vi "ArgoBot_Write.vi"(4 "GPIO 3 Write":dbl, 6 "GPIO 2 Write":dbl, 7 "Right Motor":dbl, 8 "Read_Cluster":T8, 9 "GPIO 1 Write":dbl, 10 "LED Write":bool, 11 "Left Motor":dbl) -> (3 "Write Cluster":T7)   [LabVIEW 2016, in "ArgoBotLib.lvlib"]
uses:
  ArgoBotLib.lvlib
  <vilib>/MakerHub/LINX/Private/Type Defs/LINX Ref.ctl
  <vilib>/MakerHub/LINX/Private/Type Defs/Platform.ctl
  <vilib>/MakerHub/LINX/Private/Type Defs/Interface.ctl
  <vilib>/MakerHub/LINX/Private/Device/Type Defs/LINX Device Config.ctl
  <vilib>/MakerHub/LINX/Private/Device/Type Defs/TCP Config.ctl
  <vilib>/MakerHub/LINX/Private/Device/Type Defs/Channels.ctl
  <vilib>/MakerHub/LINX/LMH-LINX.lvlib
  <vilib>/MakerHub/LINX/Private/Device/Device.lvlib
panel:
  # "ArgoBot  Write"
  # "This vi writes the GPIO channels"
  # "Inputs"
  # "Outputs"
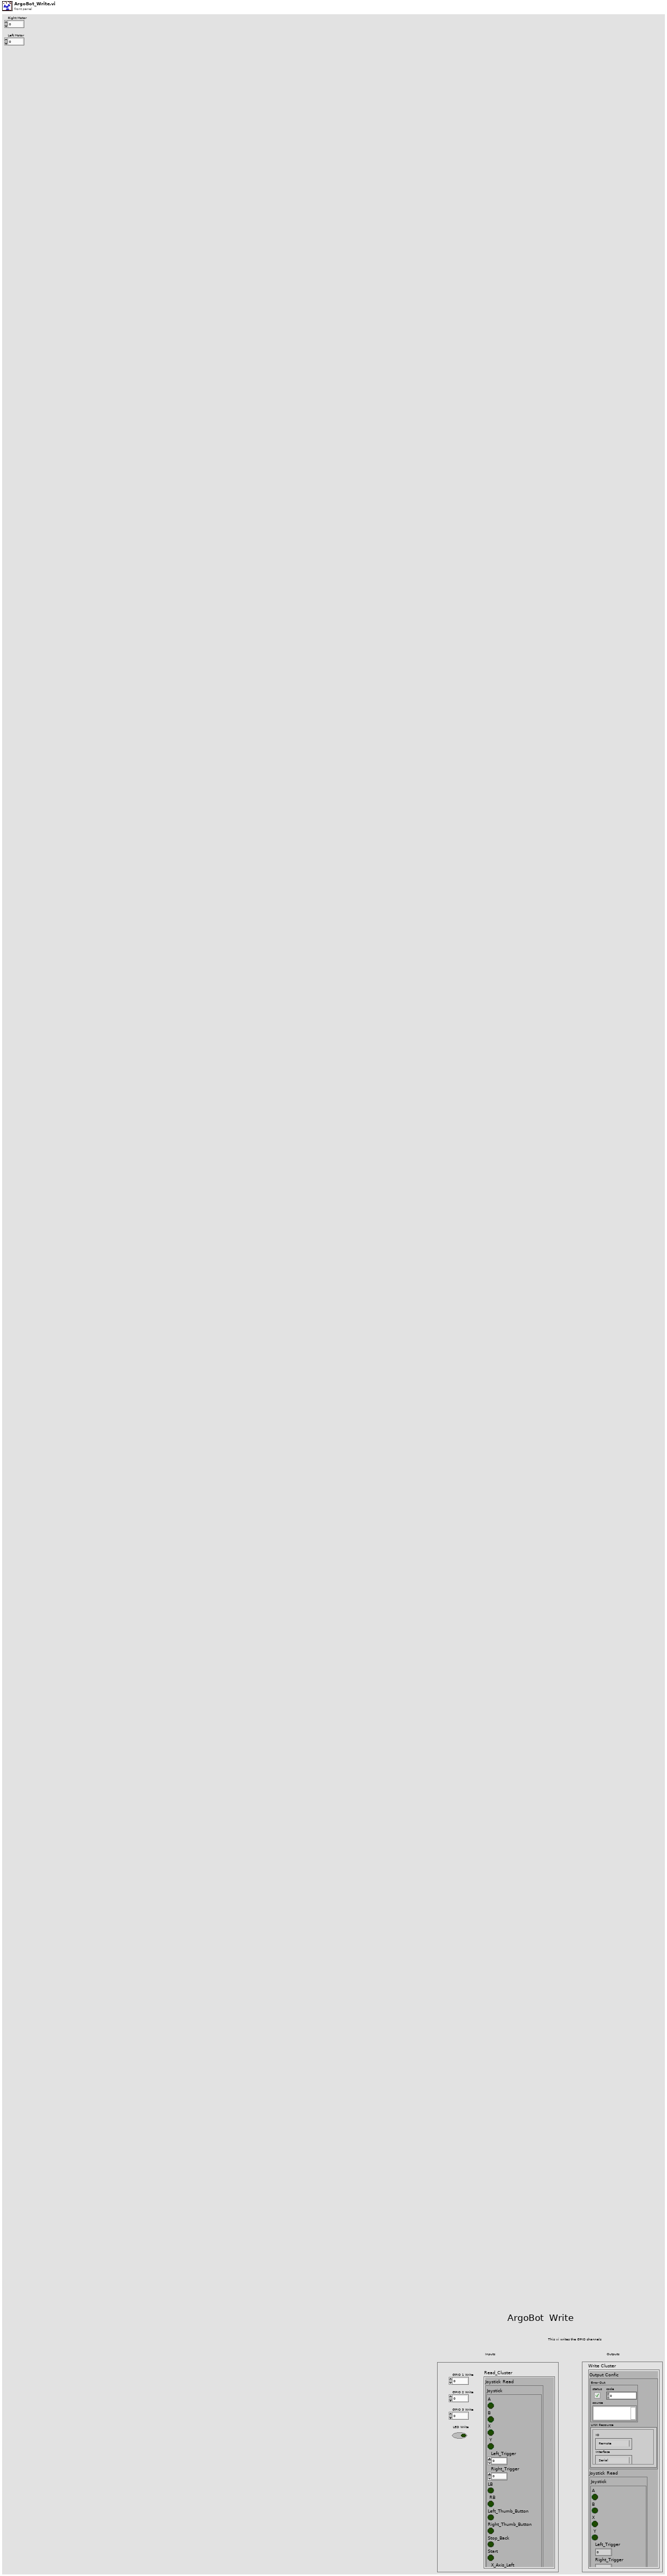
[diagram p1: front panel]
types:
  T1 = typedef "LMH-LINX.lvlib/LINX Ref.ctl" = cluster{"IO":T2, "Interface":T3, "LINX Device Config":T4}
  T2 = typedef "LMH-LINX.lvlib/Platform.ctl" = enum16{"Remote", "Local"}
  T3 = typedef "LMH-LINX.lvlib/Interface.ctl" = enum16{"Serial", "TCP"}
  T4 = typedef "LMH-LINX.lvlib/Device.lvlib/LINX Device Config.ctl" = cluster{"Interface":T3, "COM Port":refnum<visa-resource-name>, "TCP Configuration":T5, "Device Family":u8, "Device ID":u8, "Device Name":string, "TCP Ref":refnum<k5>, "Channels":T6}
  T5 = typedef "LMH-LINX.lvlib/Device.lvlib/TCP Config.ctl" = cluster{"IP Address":string, "Port":u16}
  T6 = typedef "LMH-LINX.lvlib/Channels.ctl" = cluster{"DI":u8[], "DO":u8[], "AI":u8[], "AO":u8[], "PWM":u8[], "QE":u8[], "UART":u8[], "I2C 2":u8[], "SPI":u8[], "CAN":u8[], "Servo":u8[], "AI Ref (V)":dbl, "AI Resolution (Bits)":u8, "AO Ref (V)":dbl, "AO Resolution (Bits)":u8}
  T7 = cluster{"Output Confic":cluster{"Error Out":errorcluster, "LINX Resource":T1}, "Joystick Read":cluster{"Joystick":cluster{"A":bool, "B":bool, "X":bool, " Y":bool, "Left_Trigger":dbl, "Right_Trigger ":dbl, "LB":bool, " RB":bool, "Left_Thumb_Button":bool, "Right_Thumb_Button":bool, "Stop_Back":bool, "Start":bool, "X_Axis_Left":dbl, "Y_Axis_Left":dbl, "X_Axis_Right":dbl, "Y_Axis_Right":dbl}, "Joystick error out":errorcluster, "Refnum out":refnum<k1>}, "Read Config":cluster{"Read_Config":i32[], "Error Out":errorcluster, "LINX Resource 2":T1}, "Read_Value":cluster{"Analog 1":dbl, "Analog 2":dbl, "Analog 3":dbl, "Voltage":dbl, "GPIO 1 Read":bool, "GPIO 2 Read":bool, "GPIO 3 Read":bool, "Loop Rate (Hz)":u32}, "Joystick error out":errorcluster, "Linx":cluster{"LINX Ref":T1, "Error Out":errorcluster}, "Setup":cluster{"Analog 1 Config":u16, "Analog 2 Config":u16, "Analog 3 Config":u16, "GPIO 1 Config":u16, "GPIO 2 Config":u16, "GPIO 3 Config":u16, "Drive Config":u16, "Motor Mode":u16, "Battery_Config":u16, "LED Config":u16}}
  T8 = cluster{"Joystick Read":cluster{"Joystick":cluster{"A":bool, "B":bool, "X":bool, " Y":bool, "Left_Trigger":dbl, "Right_Trigger ":dbl, "LB":bool, " RB":bool, "Left_Thumb_Button":bool, "Right_Thumb_Button":bool, "Stop_Back":bool, "Start":bool, "X_Axis_Left":dbl, "Y_Axis_Left":dbl, "X_Axis_Right":dbl, "Y_Axis_Right":dbl}, "Joystick error out":errorcluster, "Refnum out":refnum<k1>}, "Read Config":cluster{"Read_Config":i32[], "Error Out":errorcluster, "LINX Resource 2":T1}, "Read_Value":cluster{"Analog 1":dbl, "Analog 2":dbl, "Analog 3":dbl, "Voltage":dbl, "GPIO 1 Read":bool, "GPIO 2 Read":bool, "GPIO 3 Read":bool, "Loop Rate (Hz)":u32}, "Joystick error out":errorcluster, "Linx":cluster{"LINX Ref":T1, "Error Out":errorcluster}, "Setup":cluster{"Analog 1 Config":u16, "Analog 2 Config":u16, "Analog 3 Config":u16, "GPIO 1 Config":u16, "GPIO 2 Config":u16, "GPIO 3 Config":u16, "Drive Config":u16, "Motor Mode":u16, "Battery_Config":u16, "LED Config":u16}}
  T9 = cluster{"Error Out":errorcluster, "LINX Resource":T1}
  T10 = cluster{"Joystick":cluster{"A":bool, "B":bool, "X":bool, " Y":bool, "Left_Trigger":dbl, "Right_Trigger ":dbl, "LB":bool, " RB":bool, "Left_Thumb_Button":bool, "Right_Thumb_Button":bool, "Stop_Back":bool, "Start":bool, "X_Axis_Left":dbl, "Y_Axis_Left":dbl, "X_Axis_Right":dbl, "Y_Axis_Right":dbl}, "Joystick error out":errorcluster, "Refnum out":refnum<k1>}
  T11 = cluster{"Read_Config":i32[], "Error Out":errorcluster, "LINX Resource 2":T1}
  T12 = cluster{"Analog 1":dbl, "Analog 2":dbl, "Analog 3":dbl, "Voltage":dbl, "GPIO 1 Read":bool, "GPIO 2 Read":bool, "GPIO 3 Read":bool, "Loop Rate (Hz)":u32}
  T13 = cluster{"Analog 1 Config":u16, "Analog 2 Config":u16, "Analog 3 Config":u16, "GPIO 1 Config":u16, "GPIO 2 Config":u16, "GPIO 3 Config":u16, "Drive Config":u16, "Motor Mode":u16, "Battery_Config":u16, "LED Config":u16}
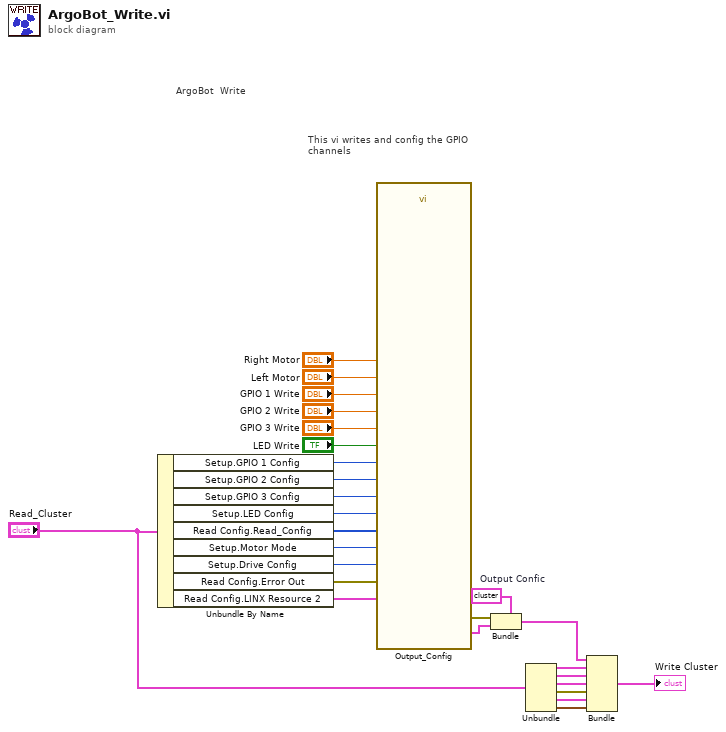
[diagram p0: block diagram]
diagram:
  w20 = T9 {"Error Out"={"status"=FALSE, "code"=0, "source"=""}, "LINX Resource"={"IO"=enum."Remote", "Interface"=enum."Serial", "LINX Device Config"={"Interface"=enum."Serial", "COM Port"="", "TCP Configuration"={"IP Address"="", "Port"=0}, "Device Family"=0, "Device ID"=0, "Device Name"="", "TCP Ref"=refnum, "Channels"={"DI"=[], "DO"=[], "AI"=[], "AO"=[], "PWM"=[], "QE"=[], "UART"=[], "I2C 2"=[], "SPI"=[], "CAN"=[], "Servo"=[], "AI Ref (V)"=0.0, "AI Resolution (Bits)"=0, "AO Ref (V)"=0.0, "AO Resolution (Bits)"=0}}}}  # Output Confic
  # "This vi writes and config the GPIO channels"
  # "ArgoBot  Write"
  n1 = Unbundle By Name("Read_Cluster") -> ("Setup.GPIO 1 Config"=w12:u16, "Setup.GPIO 2 Config"=w11:u16, "Setup.GPIO 3 Config"=w10:u16, "Setup.LED Config"=w9:u16, "Read Config.Read_Config"=w8:i32[], "Setup.Motor Mode"=w7:u16, "Setup.Drive Config"=w6:u16, "Read Config.Error Out"=w5:errorcluster, "Read Config.LINX Resource 2"=w4:T1)
  n2 = call "Output_Config.vi"("Drive Config"=w6, "Right Motor"="Right Motor", "Left Motor"="Left Motor", "LED Config"=w9, "Read_Config"=w8, "Motor Mode"=w7, "GPIO 1 Config"=w12, "GPIO 2 Config"=w11, "GPIO 3 Config"=w10, "GPIO 1 Write"="GPIO 1 Write", "GPIO 2 Write"="GPIO 2 Write", "GPIO 3 Write"="GPIO 3 Write", "LINX Resource"=w4, "LED Write"="LED Write", "Error In"=w5) -> ("Error Out"=w18:errorcluster, "LINX Resource"=w19:T1)  [unwired: 3 in]
  n3 = Bundle(cluster=w20, "Error Out"=w18, "LINX Resource"=w19) -> (w21:T9)
  n4 = Unbundle("Read_Cluster") -> ("Joystick Read"=w22:T10, "Read Config"=w23:T11, "Read_Value"=w24:T12, "Joystick error out"=w25:errorcluster, "Linx"=w26:cluster{"LINX Ref":T1, "Error Out":errorcluster}, "Setup"=w27:T13)
  n5 = Bundle("Output Confic"=w21, "Joystick Read"=w22, "Read Config"=w23, "Read_Value"=w24, "Joystick error out"=w25, "Linx"=w26, "Setup"=w27) -> (→"Write Cluster":T7)  [unwired: 1 in]
